vi "Set Events.vi"(7 "Dev Actor in":refnum<class "Dev Actor.lvclass">, 9 "Dev Actor Refs":T1, 10 "Dev Actor Events":T2) -> (5 "Dev Actor out":refnum<class "Dev Actor.lvclass">)   [LabVIEW 2021, in "Dev Actor.lvlib" / "Dev Actor.lvclass"]
uses:
  Dev Actor.lvclass
  Dev Actor.lvclass/Dev Actor.ctl
  Dev Actor Events.ctl
  Dev Actor Refs.ctl
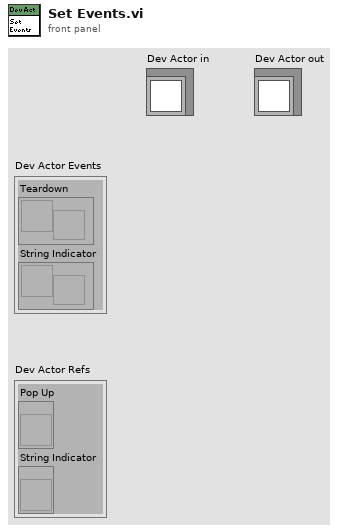
[diagram p1: front panel]
types:
  T1 = typedef "Dev Actor Refs.ctl" = cluster{"Pop Up":refnum<vi>, "String Indicator":refnum<vi>}
  T2 = typedef "Dev Actor Events.ctl" = cluster{"Teardown":refnum<user-event>, "String Indicator":refnum<user-event>}
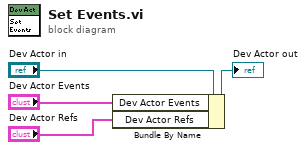
[diagram p0: block diagram]
diagram:
  n1 = Bundle By Name(cluster="Dev Actor in", "Dev Actor Events"="Dev Actor Events", "Dev Actor Refs"="Dev Actor Refs") -> (→"Dev Actor out":refnum<class "Dev Actor.lvclass">)
